vi "multi1.vi"() -> ()   [LabVIEW 2020]
uses:
  <instrlib>/_niInstr/DSP/v1/Shared/Public/IQ Data.ctl
  <vilib>/rvi/IPIntegrationNode/IPINode_Typedef/niFpgaIPINodeSupportedFamilies.ctl
  <vilib>/rvi/Emulation/niFpgaGetClockAttributes.vi
  <vilib>/rvi/Emulation/niFpgaSctlEmulationGetInTimedLoop.vi
  <vilib>/rvi/Emulation/niFpgaEmulationReportErrorSimple.vi
  <instrlib>/_niInstr/DSP/v1/FPGA/Public/Sub VIs/Frequency Shift/Frequency Shift - 1 spc.vi
  <vilib>/rvi/IPIntegrationNode/IPINode_Utilities/niFpgaIPINodeSimCore.vi
  <vilib>/rvi/Emulation/niFpgaCriticalErrorInLSC.vi
  <instrlib>/_niInstr/DSP/v1/XNodes/Public/Frequency Shift/niInstr DSP v1 Frequency Shift FPGA.xnode
  <vilib>/rvi/FXPMathLib/FxpMul/XNode/nifxpmath_Multiplier.xnode
  <vilib>/rvi/IPIntegrationNode/IPINode_Xnode/niFpgaIPINode.xnode
  MULTIPLY/MULTIPLY.srcs/sources_1/new/IP_BlockSimFiles/xsim.dir/multiwrapper/xsimk81D7C81F6B8041B1B6096E826D8D5E25.dll
  <vilib>/rvi/Analysis/measure/butterworth/XNode/niFpgaButterworthFilter.xnode
  <instrlib>/_niInstr/DSP/v1/Shared/niInstr DSP v1 Shared.lvlib
  <instrlib>/_niInstr/DSP/v1/FPGA/niInstr DSP v1 FPGA.lvlib
  <vilib>/rvi/FXPMathLib/sim/FxpSim.dll
panel:
  out "appended array 2":cluster{sgl, sgl}(graph)={50523456.0, 49561028.0}
  out "appended array":cluster{sgl, sgl}(graph)={4840.0, 10710.0}
  in  "frequency(kHz) 2":fxp<+,32,16>=10.0
  in  "frequency(kHz)":fxp<+,32,16>=20.0
  in  "amplitude":fxp<+/-,16,16>=16383.0
  in  "stop":bool
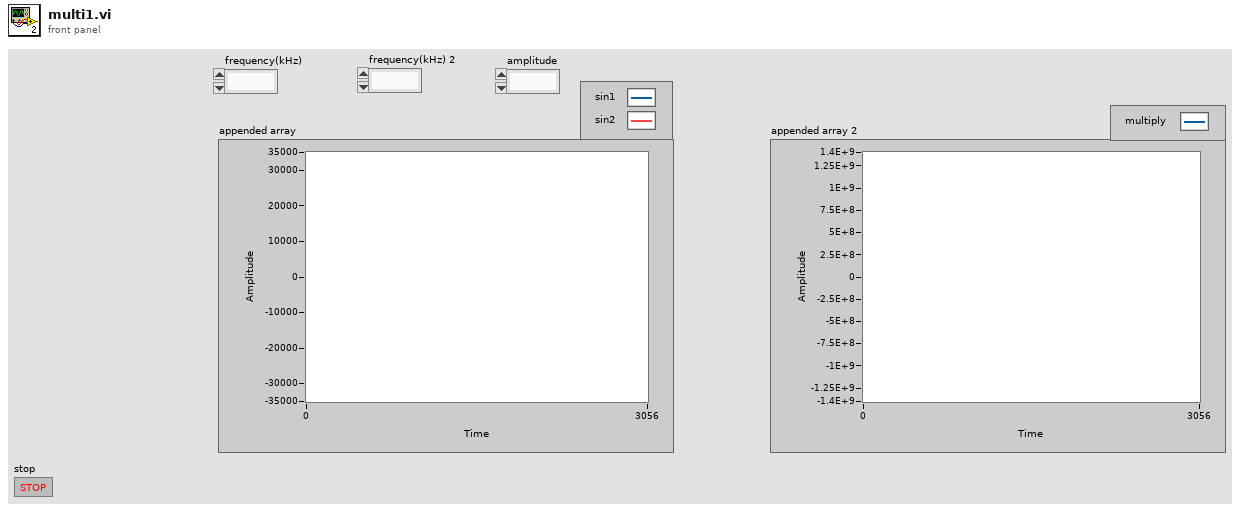
[diagram p1: front panel]
types:
  T1 = typedef "niFpgaIPINodeSupportedFamilies.ctl" = cluster{"unlimited?":bool, "supported targets":string[]}
  T2 = typedef "niInstr DSP v1 Shared.lvlib/IQ Data.ctl" = cluster{"I":fxp<+/-,18,1>, "Q":fxp<+/-,18,1>, "overflow":bool}
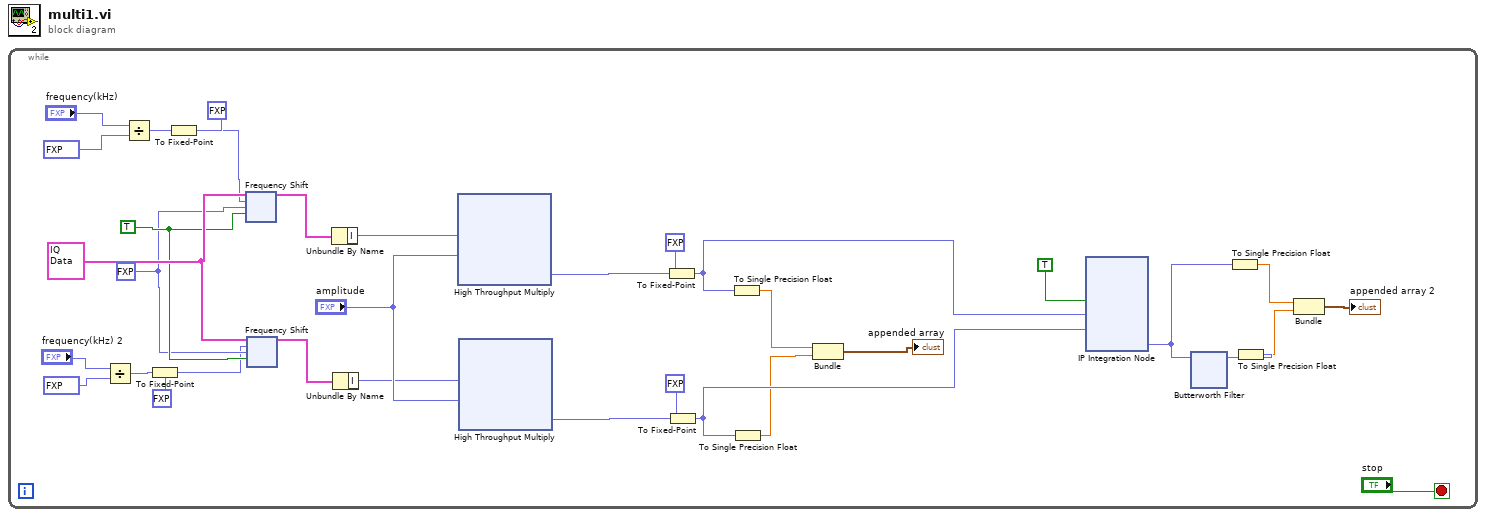
[diagram p0: block diagram]
diagram:
  n1 = while {
    stop <- "stop" stop-if-true
    w22 = T2 {"I"=0.9999923706054688, "Q"=0.0, "overflow"=FALSE} ("data in")
    w21 = TRUE ("input valid")
    w20 = fxp<+/-,21,0> 0.0 ("phase")
    n2 = Divide(x="frequency(kHz) 2", y=fxp<+,32,16> 40000.0 ("frequency (periods/tick)")) -> (x/y=w8:fxp<+,64,32>)
    n3 = Divide(x="frequency(kHz)", y=fxp<+,32,16> 40000.0 ("frequency (periods/tick)")) -> (x/y=w13:fxp<+,64,32>)
    n4 = To Fixed-Point(fixed-point type=fxp<+/-,48,0> 0.0 ("frequency shift"), number=w8) -> (fixed-point=w7:fxp<+/-,48,0>)
    n5 = To Fixed-Point(fixed-point type=fxp<+/-,48,0> 0.0 ("frequency shift"), number=w13) -> (fixed-point=w12:fxp<+/-,48,0>)
    n6 = xnode "Frequency Shift"("data in"=w22, "frequency shift"=w12, "phase"=w20, "input valid"=w21) -> ("data out"=w32:T2)  [unwired: 2 in, 2 out]
    n7 = xnode "Frequency Shift"("data in"=w22, "frequency shift"=w7, "phase"=w20, "input valid"=w21) -> ("data out"=w25:T2)  [unwired: 2 in, 2 out]
    n8 = Unbundle By Name(w32) -> ("I"=w31:fxp<+/-,18,1>)
    n9 = Unbundle By Name(w25) -> ("I"=w17:fxp<+/-,18,1>)
    n10 = xnode "High Throughput Multiply"("x"=w31, "y"="amplitude") -> ("x*y"=w30:fxp<+/-,34,17>)
    n11 = xnode "High Throughput Multiply"("x"=w17, "y"="amplitude") -> ("x*y"=w26:fxp<+/-,34,17>)
    n12 = To Fixed-Point(fixed-point type=fxp<+/-,16,16> 0.0, number=w30) -> (fixed-point=w28:fxp<+/-,16,16>)
    n13 = To Fixed-Point(fixed-point type=fxp<+/-,16,16> 0.0, number=w26) -> (fixed-point=w24:fxp<+/-,16,16>)
    n14 = To Single Precision Float(number=w28) -> (single precision float=w6:sgl)
    n15 = To Single Precision Float(number=w24) -> (single precision float=w5:sgl)
    n16 = Bundle(w6, w5) -> (→"appended array":cluster{sgl, sgl})  [unwired: 1 in]
    n17 = xnode "IP Integration Node"("cEn"=TRUE, "sig_i_1"=w28, "sig_i_2"=w24) -> ("sig_o"=w19:fxp<+/-,32,32>)
    n18 = xnode "Butterworth Filter"("input data"=w19) -> ("output data"=w18:fxp<+/-,32,32>)  [unwired: 2 in]
    n19 = To Single Precision Float(number=w19) -> (single precision float=w2:sgl)
    n20 = To Single Precision Float(number=w18) -> (single precision float=w1:sgl)
    n21 = Bundle(w2, w1) -> (→"appended array 2":cluster{sgl, sgl})  [unwired: 1 in]
  }
